vi "Read MagFieldTable.vi"(8 "error in (no error)":errorcluster, 11 "MagFieldTable in":refnum<class "MagFieldTable.lvclass">) -> (0 "error out":errorcluster, 2 "MagFieldTable":string[][](table), 3 "MagFieldTable out":refnum<class "MagFieldTable.lvclass">)   [LabVIEW 2018, in "MagFieldTable.lvclass"]
uses:
  MagFieldTable.lvclass
  MagFieldTable.lvclass/MagFieldTable.ctl
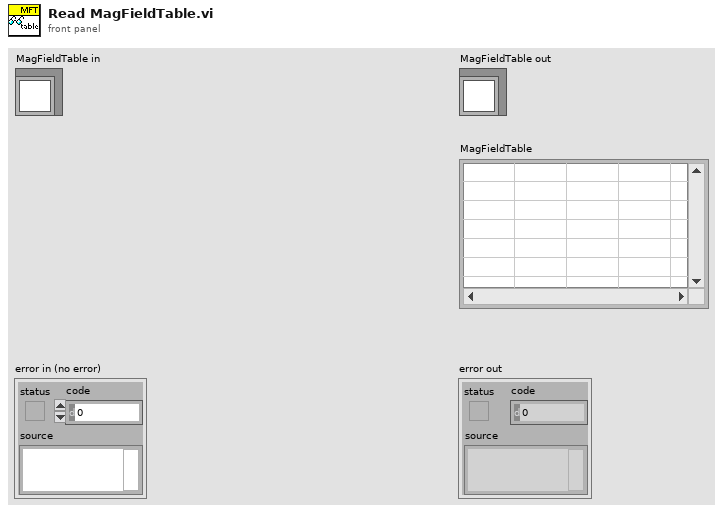
[diagram p1: front panel]
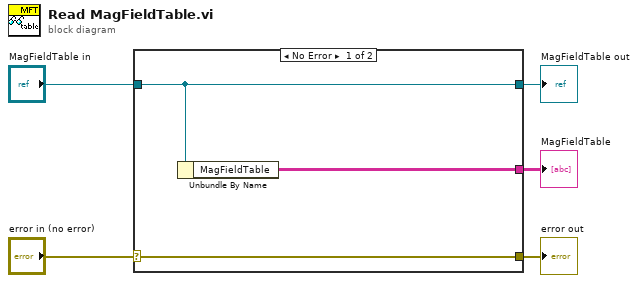
[diagram p0: block diagram]
diagram:
  n1 = case shown="No Error" "error in (no error)" {
    selector: "error in (no error)" -> [w8 w9]
    tunnel: [w8 w9] -> w4
    tunnel: [w7 w10] -> w2
    tunnel: "MagFieldTable in" -> [w7 w10]
    tunnel: [w6 _] -> w1
    frame No Error {
      n2 = Unbundle By Name(w7) -> ("MagFieldTable"=w6:string[][])
    }
    frame Error {
    }
  }
  "error out" <- w4
  "MagFieldTable out" <- w2
  "MagFieldTable" <- w1
